vi "NGTS_ - Sort PID Tags into Sets and Gain Schedules .vi"(8 "error in":errorcluster, 11 "Tags":string[](array[string])=["PID_001_SP", "PID_001_PV", "PID_001_OUTH", "PID_001_OUTL", "PID_001_MODE", "PID_001_GSV", "PID_001_P1", "PID_001_I1", "PID_001_D1", "PID_001_GSM1", "PID_001_P2", "PID_001_I2", "PID_001_D2", "PID_001_GSM2", "PID_001_SPMAX", "PID_001_SPMIN", "PID_002_SP", "PID_002_PV", "PID_002_OUTH", "PID_002_OUTL", "PID_002_MODE", "PID_002_GSV", "PID_002_P1", "PID_002_I1", "PID_002_D1", "PID_002_GSM1", "PID_002_P2", "PID_002_I2", "PID_002_D2", "PID_002_GSM2", "PID_002_P3", "PID_002_I3", "PID_002_D3", "PID_002_GSM3", "PID_002_SPMAX", "PID_002_SPMIN", "PID_003_SP", "PID_003_PV", "PID_003_OUTH", "PID_003_OUTL", "PID_003_MODE", "PID_003_GSV", "PID_003_P1", "PID_003_I1", "PID_003_D1", "PID_003_GSM1", "PID_003_P2", "PID_003_I2", "PID_003_D2", "PID_003_GSM2", "PID_003_SPMAX", "PID_003_SPMIN"]) -> (0 "error out":errorcluster, 1 "Gain Set Checks":T1(array[cluster]), 3 "PID Tag Sets":T2[](array[typedef]), 5 "PID Loops":i32)   [LabVIEW 2010]
doc: "This VI filters a system Tag list into sets of PID parameters and Gain Scheduling sets for each PID loop. It checks to see that each PID has all the correct parameters and that each Gain set has the correct number of parameters.\n\nThe standard PID input tag set is (example is loop# 001):\n\nPID_001_SP Setpoint\nPID_001_PV Process Variable\nPID_001_SPMAX Setpoint Max\nPID_001_SPMIN Setpoint Min\nPID_001_GSV Gain Schedule Variable\nPID_001_OUTH Output High Limit\nPID_001_OUTL Output Low Limit\nPID_001_MODE Mode: Auto (T) || Manaual (F)\nPID_001_MAN Value out in Manual Mode\n\nPlus at least one Gain Schedule Set of:\nPID_001_Pm Proportional\nPID_001_Im Integral\nPID_001_Dm Derivative\nPID_001_GSVMm GSVMax\n\nWhere m is the Gain Set number. The GSV is thresholded against the set of GSVMs to determine which Gain Set to use on a given loop iteration.\n\n2008_01_09 Mike Ashe\nmichael.ashe@imaginatics.net\nCell: 860-961-0876"
uses:
  Controls/NGTS_PID Loop Tag and Gain Set.ctl
  <userlib>/_OpenG.lib/array/array.llb/Filter 1D Array (String)__ogtk.vi
panel:
  out "Gain Sets Ok?":bool
  out "Array of Strings":string[](array[string])
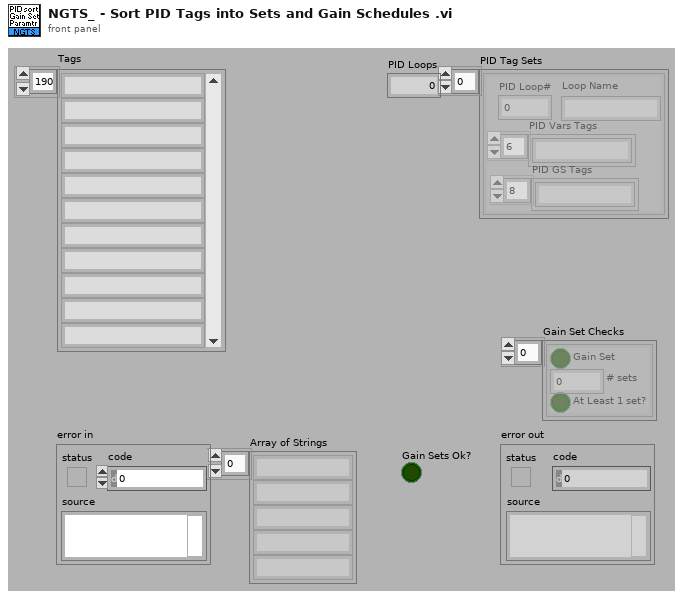
[diagram p1: front panel]
types:
  T1 = cluster{"Gain Set":bool, "# sets":i32, "At Least 1 set?":bool}[]
  T2 = typedef "NGTS_PID Loop Tag and Gain Set.ctl" = cluster{"PID Loop#":i32, "PID Vars Tags":string[], "PID GS Tags":string[], "Loop Name":string}
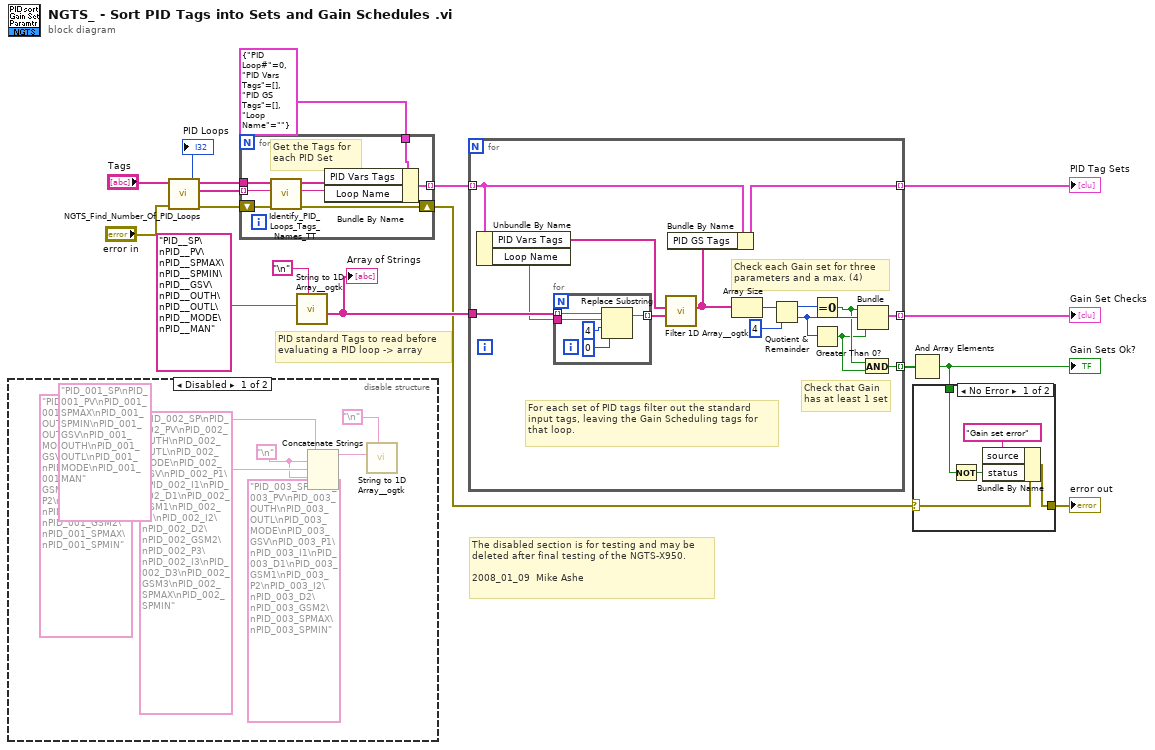
[diagram p0: block diagram]
diagram:
  # "PID standard Tags to read before\nevaluating a PID loop -> array"
  # "The disabled section is for testing and may be\ndeleted after final testing of the NGTS-X950.\n\n2008_01_09  Mike Ashe"
  n1 = disable-structure shown="Disabled" {
    frame Disabled {
      (unwired) "PID_001_SP\nPID_001_PV\nPID_001_SPMAX\nPID_001_SPMIN\nPID_001_GSV\nPID_001_OUTH\nPID_001_OUTL\nPID_001_MODE\nPID_001_MAN"
      w20 = "\n"
      n2 = Concatenate Strings("PID_001_SP\nPID_001_PV\nPID_001_OUTH\nPID_001_OUTL\nPID_001_MODE\nPID_001_GSV\nPID_001_P1\nPID_001_I1\nPID_001_D1\nPID_001_GSM1\nPID_001_P2\nPID_001_I2\nPID_001_D2\nPID_001_GSM2\nPID_001_SPMAX\nPID_001_SPMIN", w20, "PID_002_SP\nPID_002_PV\nPID_002_OUTH\nPID_002_OUTL\nPID_002_MODE\nPID_002_GSV\nPID_002_P1\nPID_002_I1\nPID_002_D1\nPID_002_GSM1\nPID_002_P2\nPID_002_I2\nPID_002_D2\nPID_002_GSM2\nPID_002_P3\nPID_002_I3\nPID_002_D3\nPID_002_GSM3\nPID_002_SPMAX\nPID_002_SPMIN", w20, "PID_003_SP\nPID_003_PV\nPID_003_OUTH\nPID_003_OUTL\nPID_003_MODE\nPID_003_GSV\nPID_003_P1\nPID_003_I1\nPID_003_D1\nPID_003_GSM1\nPID_003_P2\nPID_003_I2\nPID_003_D2\nPID_003_GSM2\nPID_003_SPMAX\nPID_003_SPMIN") -> (w18:string)
      n3 = call <userlib>:"String to 1D Array__ogtk.vi"("delimiter (Tab)"="\n", "string"=w18) -> ()  [unwired: 9 in, 1 out]
    }
    frame Enabled {
    }
  }
  n4 = call "NGTS_Find_Number_Of_PID_Loops.vi"("error in"="error in", "Tags"="Tags") -> ("error out"=w17:errorcluster, "PID Loop Names"=w15:string[], "PID Tags"=w16:string[], "PID Loops"=→"PID Loops":i32)  [unwired: 6 in]
  n5 = for {
    tunnel: w16 -> [w30]
    tunnel: w15 -> [w29] mode=indexing
    tunnel: T2 {"PID Loop#"=0, "PID Vars Tags"=[], "PID GS Tags"=[], "Loop Name"=""} ("PID Tag Set") -> [w28]
    tunnel: [w25] -> w12 mode=indexing
    shift-right: [w24] -> w3
    shift-left: w17 -> [w31]
    # "Get the Tags for \neach PID Set"
    n6 = call "Identify_PID_Loops_Tags_Names_TT.vi"("error in"=w31, "PID_Loop Names"=w29, "Tags"=w30) -> ("error out"=w24:errorcluster, "PID_Loop Names Out"=w26:string, "PID Tag Set"=w27:string[])  [unwired: 6 in]
    n7 = Bundle By Name(cluster=w28, "PID Vars Tags"=w27, "Loop Name"=w26) -> (w25:T2)
  }
  n8 = call <userlib>:"String to 1D Array__ogtk.vi"("delimiter (Tab)"="\n", "string"="PID__SP\nPID__PV\nPID__SPMAX\nPID__SPMIN\nPID__GSV\nPID__OUTH\nPID__OUTL\nPID__MODE\nPID__MAN") -> ("Array of Strings"=w11:string[])  [unwired: 9 in]
  "Array of Strings" <- w11
  n9 = for {
    tunnel: w12 -> [w45] mode=indexing
    tunnel: w11 -> [w43]
    tunnel: [w44] -> w1 mode=indexing
    tunnel: [w36] -> w9 mode=indexing
    tunnel: [w33] -> w8 mode=indexing
    # "Check that Gain\nhas at least 1 set"
    # "Check each Gain set for three\nparameters and a max. (4)"
    # "For each set of PID tags filter out the standard\ninput tags, leaving the Gain Scheduling tags for\nthat loop."
    n10 = Unbundle By Name(w45) -> ("PID Vars Tags"=w46:string[], "Loop Name"=w32:string)
    n11 = for {
      tunnel: w43 -> [w51] mode=indexing
      tunnel: [w50] -> w42 mode=indexing
      tunnel: w32 -> [w47]
      n12 = Replace Substring(2:0 ("length (len. of substring)"), 3:4 ("offset (0)"), 4:w47, 5:w51) -> (1:w50:string)  [unwired: 1 out]
    }
    n13 = call-poly <userlib>:"Filter 1D Array__ogtk.vi"("items to filter"=w42, "array"=w46) -> ("filtered array"=w41:string[])  [unwired: 4 in, 1 out]
    n14 = Bundle By Name(cluster=w45, "PID GS Tags"=w41) -> (w44:T2)
    n15 = Array Size(array=w41) -> (size(s)=w40:i32)
    n16 = Quotient & Remainder(x=w40, y=4) -> (x-y*floor(x/y)=w38:i32, floor(x/y)=w37:i32)
    n17 = Equal To 0?(x=w38) -> (x = 0?=w35:bool)
    n18 = Greater Than 0?(x=w37) -> (x > 0?=w34:bool)
    n19 = Bundle(w35, w37, w34) -> (w36:cluster{bool, i32, bool})  [unwired: 1 in]
    n20 = And(x=w35, y=w34) -> (x .and. y?=w33:bool)
  }
  "PID Tag Sets" <- w1
  "Gain Set Checks" <- w9
  n21 = And Array Elements(Boolean array=w8) -> (logical AND=w5:bool)
  "Gain Sets Ok?" <- w5
  n22 = case shown="No Error" w3 {
    selector: w3 -> [w52 w57]
    tunnel: w5 -> [w56 _]
    tunnel: [w54 w57] -> w4
    frame No Error {
      n23 = Not(x=w56) -> (.not. x?=w55:bool)
      n24 = Bundle By Name(cluster=w52, "source"="Gain set error", "status"=w55) -> (w54:errorcluster)
    }
    frame Error {
    }
  }
  "error out" <- w4
